vi "handleIncomingMessages.vi"(7 "onIncomingMessagingError":refnum<class "Command.lvclass">, 8 "error in (no error)":errorcluster, 9 "commandToProcessEvent":T1, 11 "UserEventBasedController in":refnum<class "UserEventBasedController.lvclass">) -> (0 "error out":errorcluster, 3 "UserEventBasedController out":refnum<class "UserEventBasedController.lvclass">)   [LabVIEW 2015, in "UserEventBasedController.lvclass"]
uses:
  ComponentTemplateCore/ComponentModel/ComponentModel/UserEventBasedController/UserEventBasedController.lvclass
  ComponentTemplateCore/ComponentModel/ComponentModel/CommandEvent/CommandEvent.lvclass
  ComponentTemplateCore/ComponentModel/ComponentModel/Rendezvous/Rendezvous.lvclass
  ComponentTemplateCore/ComponentModel/ComponentModel/InternalSignals/stop.vi
  ComponentTemplateCore/ComponentModel/ComponentModel/InternalSignals/InternalSignalsGlobals.lvlib
  ComponentTemplateCore/ComponentModel/ComponentModel/Command/Command.lvclass
  ComponentTemplateCore/ComponentModel/ComponentModel/InternalSignals/error.vi
  ComponentTemplateCore/ComponentModel/ComponentModel/InternalSignals/clearMessagingError.vi
  ComponentTemplateCore/ComponentModel/ComponentModel/MiddlewareProcessEvent/MiddlewareProcessEvent.lvclass
  ComponentTemplateCore/ComponentModel/ComponentModel/Typedefs/CommandToProcessEvent.ctl
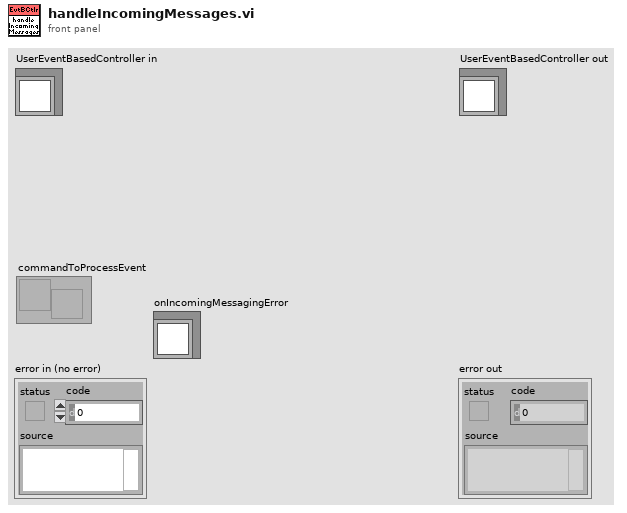
[diagram p1: front panel]
types:
  T1 = typedef "CommandToProcessEvent.ctl" = refnum<user-event>
  T2 = typedef "HeartbeatConfig.ctl" = cluster{"Heartbeat Interval (s)":dbl, "Heartbeat Timeout (s)":dbl}
  T3 = typedef "EXATypedefs.lvlib/CommandEvents.ctl" = cluster{"command":refnum<user-event>}
  T4 = typedef "MiddlewareProcessEvents.ctl" = cluster{"disconnect":refnum<user-event>, "error":refnum<user-event>}
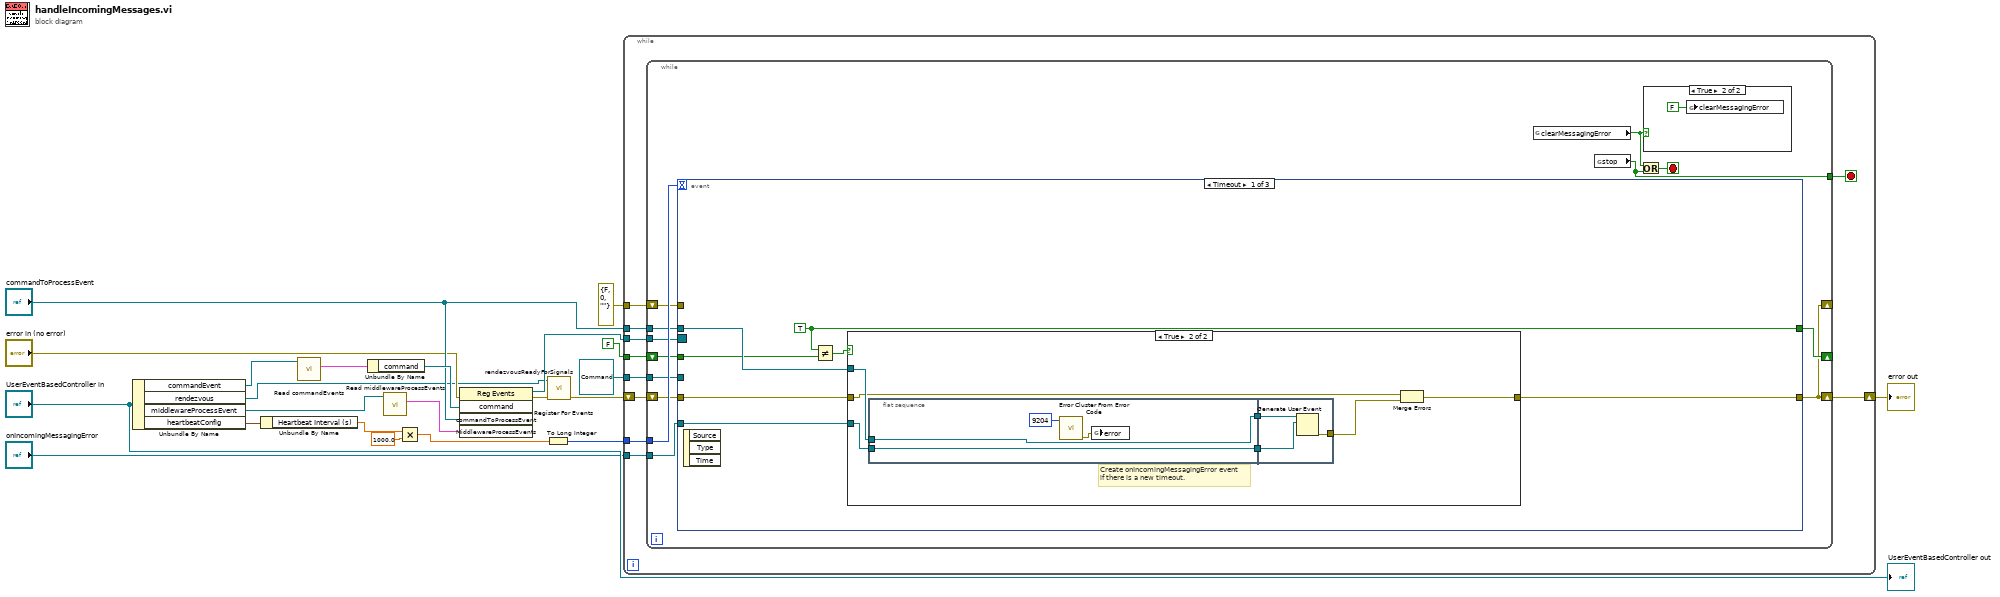
[diagram p0: block diagram]
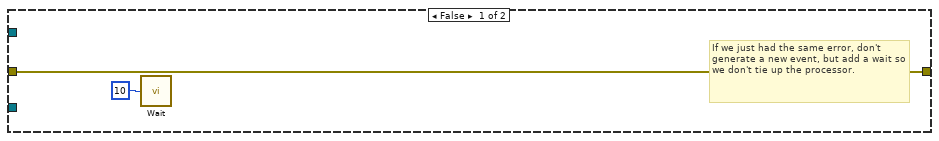
[diagram p3: hidden frame]
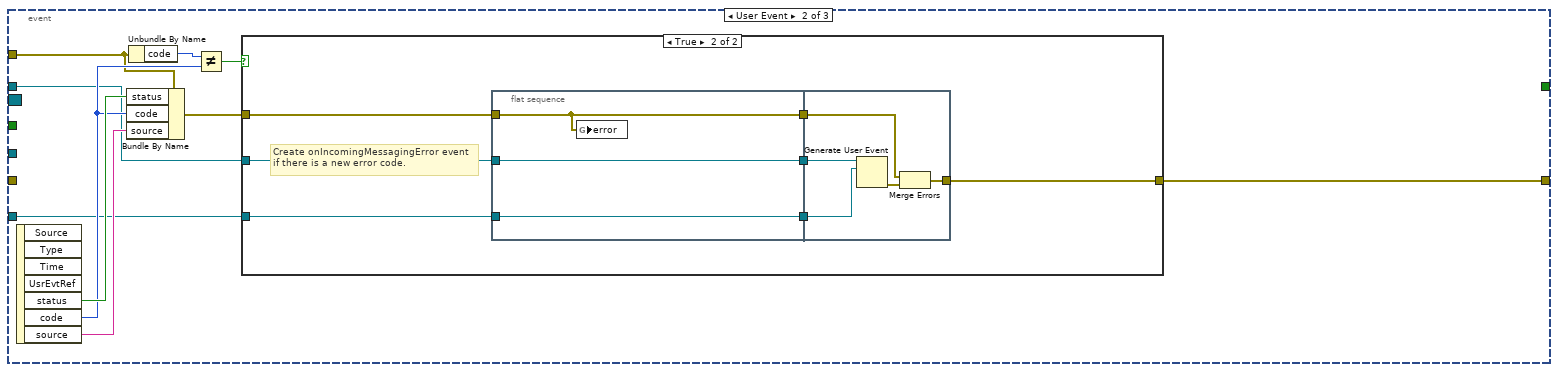
[diagram p4: hidden frame]
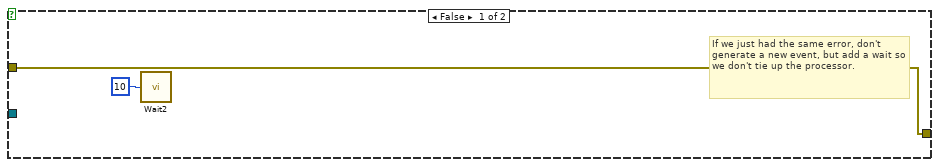
[diagram p5: hidden frame]
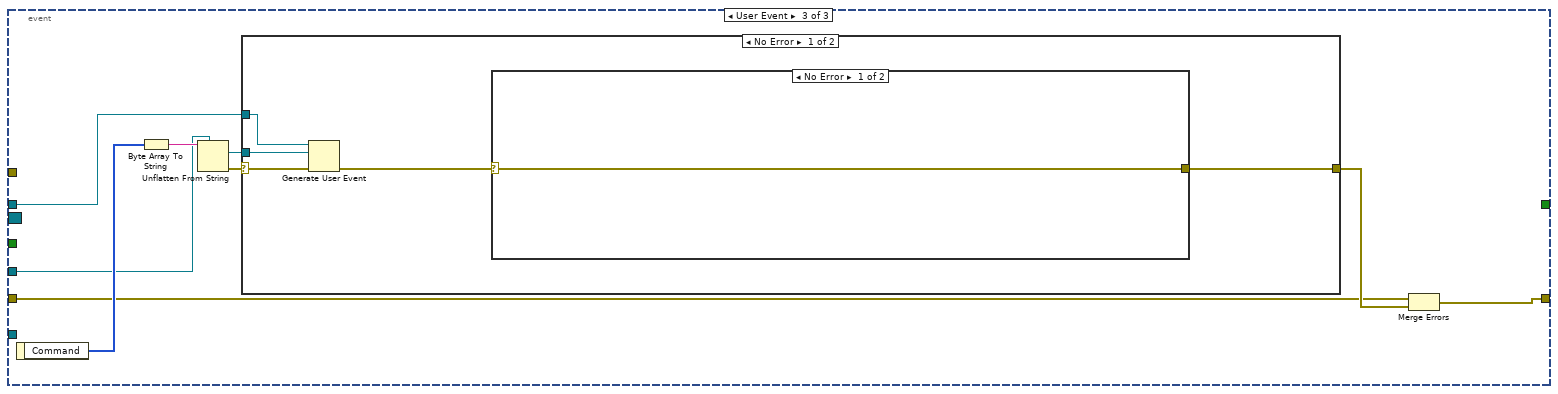
[diagram p6: hidden frame]
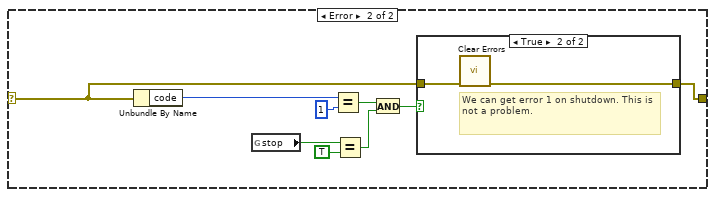
[diagram p7: hidden frame]
diagram:
  n1 = Unbundle By Name("UserEventBasedController in") -> ("commandEvent"=w5:refnum<class "CommandEvent.lvclass">, "rendezvous"=w4:refnum<class "Rendezvous.lvclass">, "middlewareProcessEvent"=w3:refnum<class "MiddlewareProcessEvent.lvclass">, "heartbeatConfig"=w2:T2)
  n2 = Unbundle By Name(w2) -> ("Heartbeat Interval (s)"=w20:dbl)
  n3 = call "Read commandEvents.vi"("CommandEvent in"=w5) -> ("CommandEvents"=w22:T3)  [unwired: 9 in, 1 out]
  n4 = Unbundle By Name(w22) -> ("command"=w21:refnum<user-event>)
  n5 = call "Read middlewareProcessEvents.vi"("MiddlewareProcessEvent in"=w3) -> ("MiddlewareProcessEvents"=w8:T4)  [unwired: 9 in, 1 out]
  n6 = Multiply(x=w20, y=1000.0) -> (x*y=w18:dbl)
  n7 = register-events(error in="error in (no error)", w21, "commandToProcessEvent", w8) -> (reference out=w16:refnum<event-registration>, error out=w12:errorcluster)  [unwired: 1 in]
  n8 = To Long Integer(number=w18) -> (32bit integer=w17:i32)
  n9 = call "rendezvousReadyForSignals.vi"("error in (no error)"=w12, "Rendezvous in"=w4) -> ("error out"=w11:errorcluster)  [unwired: 8 in, 1 out]
  n10 = while {
    tunnel: w17 -> [w32]
    tunnel: w16 -> [w31]
    tunnel: refnum<class "Command.lvclass"> refnum ("Command.lvclass") -> [w30]
    tunnel: "commandToProcessEvent" -> [w29]
    tunnel: FALSE -> [w26]
    tunnel: "onIncomingMessagingError" -> [w25]
    tunnel: errorcluster {"status"=FALSE, "code"=0, "source"=""} ("error IO") -> [w24]
    shift-right: [w27] -> w10
    shift-left: w11 -> [w28]
    stop <- w23 stop-if-true
    n11 = while {
      tunnel: w32 -> [w45]
      tunnel: w31 -> [w44]
      tunnel: w30 -> [w43]
      tunnel: w29 -> [w42]
      shift-right: [w33] -> w27
      shift-left: w28 -> [w41]
      tunnel: w25 -> [w40]
      shift-right: [w39] -> _
      shift-left: w26 -> [w38]
      shift-right: [w33] -> _
      shift-left: w24 -> [w36]
      tunnel: [w34] -> w23
      stop <- w35 stop-if-true
      n12 = event shown="[0] Timeout" {
        selector: w44 -> [_ _ _]
        dyn-events: _ -> [_ _ _]
        timeout: w45 -> [_ _ _]
        tunnel: w43 -> [_ _ w100]
        tunnel: w42 -> [w53 w74 w99]
        tunnel: w41 -> [w52 _ w98]
        tunnel: [w51 w73 w97] -> w33
        tunnel: w40 -> [w48 w75 _]
        tunnel: [w47 _ _] -> w39
        tunnel: w38 -> [w50 _ _]
        tunnel: w36 -> [_ w72 _]
        event Timeout {
          w47 = TRUE
          n13 = event-data() -> ()  [unwired: 1 in, 3 out]
          n14 = Not Equal?(x=w47, y=w50) -> (x != y?=w49:bool)
          n15 = case shown="True" w49 {
            tunnel: [w54 w61] -> w51
            tunnel: w48 -> [_ w59]
            tunnel: w53 -> [_ w57]
            tunnel: w52 -> [w54 w56]
            frame False {
              # "If we just had the same error, don't generate a new event, but add a wait so we don't tie up the processor."
              n16 = call "Wait"("Count(mSec)"=u32 10) -> ()  [unwired: 1 out]
            }
            frame True {
              # "Create onIncomingMessagingError event if there is a new timeout."
              n17 = flat-sequence {
                tunnel: [w64] -> w60
                tunnel: w59 -> [w64]
                tunnel: [w63] -> w58
                tunnel: w57 -> [w63]
                tunnel: [w68] -> w62
                tunnel: w60 -> [w67]
                tunnel: w58 -> [w69]
                frame #0 {
                  n18 = call <vilib>:"Error Cluster From Error Code.vi"("error code (0)"=9204) -> ("error out"=w65:errorcluster)  [unwired: 8 in]
                  n19 = global write "error.vi" "error"(w65) -> ()
                }
                frame #1 {
                  n20 = Generate User Event(user event=w69, event data cluster=w67) -> (error out=w68:errorcluster)  [unwired: 2 in, 1 out]
                }
              }
              n21 = Merge Errors(w56, w62) -> (w61:errorcluster)
            }
          }
        }
        event User Event {
          n22 = event-data() -> ("status"=w79:bool, "code"=w78:i32, "source"=w77:string)  [unwired: 1 in, 4 out]
          n23 = Bundle By Name(cluster=w72, "status"=w79, "code"=w78, "source"=w77) -> (w76:errorcluster)
          n24 = Unbundle By Name(w72) -> ("code"=w71:i32)
          n25 = Not Equal?(x=w71, y=w78) -> (x != y?=w70:bool)
          n26 = case shown="True" w70 {
            tunnel: w76 -> [w81 w85]
            tunnel: w75 -> [_ w84]
            tunnel: w74 -> [_ w83]
            tunnel: [w81 w82] -> w73
            frame False {
              # "If we just had the same error, don't generate a new event, but add a wait so we don't tie up the processor."
              n27 = call "Wait2"("Count(mSec)"=u32 10) -> ()  [unwired: 1 out]
            }
            frame True {
              # "Create onIncomingMessagingError event if there is a new error code."
              n28 = flat-sequence {
                tunnel: w85 -> [w89]
                tunnel: w84 -> [w90]
                tunnel: w83 -> [w91]
                tunnel: [w91] -> w88
                tunnel: [w90] -> w87
                tunnel: [w89] -> w86
                tunnel: [w92] -> w82
                tunnel: w88 -> [w96]
                tunnel: w87 -> [w95]
                tunnel: w86 -> [w94]
                frame #0 {
                  n29 = global write "error.vi" "error"(w89) -> ()
                }
                frame #1 {
                  n30 = Generate User Event(user event=w96, event data cluster=w95) -> (error out=w93:errorcluster)  [unwired: 2 in, 1 out]
                  n31 = Merge Errors(w94, w93) -> (w92:errorcluster)
                }
              }
            }
          }
        }
        event User Event {
          n32 = event-data() -> ("Command"=w101:u8[])  [unwired: 1 in]
          n33 = Byte Array To String(unsigned byte array=w101) -> (string=w105:string)
          n34 = Unflatten From String(type=w100, binary string=w105) -> (value=w103:refnum<class "Command.lvclass">, error out=w104:errorcluster)  [unwired: 3 in, 1 out]
          n35 = case shown="No Error" w104 {
            selector: w104 -> [w108 w124]
            tunnel: w99 -> [w110 _]
            tunnel: w103 -> [w109 _]
            tunnel: [w106 w124] -> w102
            frame No Error {
              n36 = Generate User Event(user event=w110, event data cluster=w109, error in=w108) -> (error out=w107:errorcluster)  [unwired: 1 in, 1 out]
              n37 = case shown="No Error" w107 {
                selector: w107 -> [w111 w117]
                tunnel: [w111 w116] -> w106
                frame No Error {
                }
                frame Error {
                  n38 = Unbundle By Name(w117) -> ("code"=w119:i32)
                  n39 = global read "stop.vi" "stop"() -> (w120:bool)
                  n40 = Equal?(x=w119, y=1) -> (x = y?=w113:bool)
                  n41 = Equal?(x=w120, y=TRUE) -> (x = y?=w112:bool)
                  n42 = And(x=w113, y=w112) -> (x .and. y?=w114:bool)
                  n43 = case shown="True" w114 {
                    tunnel: w117 -> [w121 w123]
                    tunnel: [w121 w122] -> w116
                    frame False {
                    }
                    frame True {
                      # "We can get error 1 on shutdown. This is not a problem."
                      n44 = call <vilib>:"Clear Errors.vi"("error in (no error)"=w123) -> ("error out"=w122:errorcluster)  [unwired: 5 in, 1 out]
                    }
                  }
                }
              }
            }
            frame Error {
            }
          }
          n45 = Merge Errors(w98, w102) -> (w97:errorcluster)
        }
      }
      n46 = global read "clearMessagingError.vi" "clearMessagingError"() -> (w37:bool)
      n47 = global read "stop.vi" "stop"() -> (w34:bool)
      n48 = Or(x=w37, y=w34) -> (x .or. y?=w35:bool)
      n49 = case shown="True" w37 {
        frame False {
        }
        frame True {
          n50 = global write "clearMessagingError.vi" "clearMessagingError"(FALSE ("clearError")) -> ()
        }
      }
    }
  }
  "error out" <- w10
  "UserEventBasedController out" <- "UserEventBasedController in"
